vi "Copy Build to Shared Location.vi"(7 "Retain Build":bool, 8 "error in (no error)":errorcluster, 9 "Workspace":path, 10 "Job":string, 11 "Build Number":u32) -> (0 "error out":errorcluster)   [LabVIEW 2010]
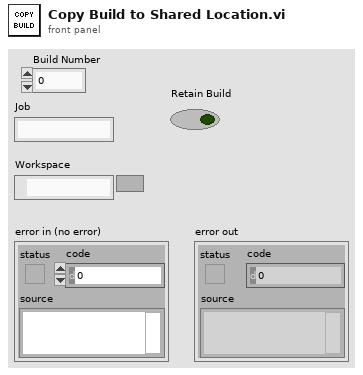
[diagram p1: front panel]
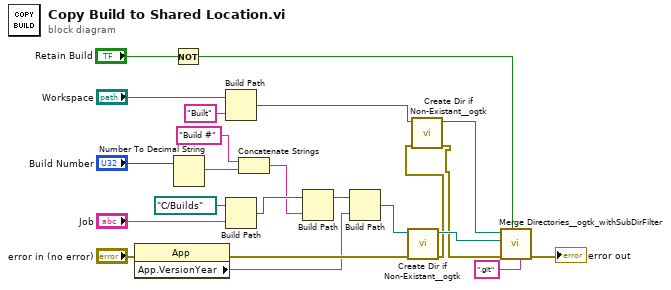
[diagram p0: block diagram]
diagram:
  n1 = property class="App"(error in="error in (no error)") -> (error out=w9:errorcluster, "App.VersionYear"=w7:string)  [unwired: 1 in, 1 out]
  n2 = Not(x="Retain Build") -> (.not. x?=w5:bool)
  n3 = Number To Decimal String(number="Build Number") -> (decimal integer string=w21:string)  [unwired: 1 in]
  n4 = Build Path(base path="Workspace", name or relative path="Built") -> (appended path=w4:path)
  n5 = Build Path(base path=path "C:/Builds", name or relative path="Job") -> (appended path=w20:path)
  n6 = Concatenate Strings("Build #", w21) -> (w8:string)
  n7 = Build Path(base path=w20, name or relative path=w8) -> (appended path=w10:path)
  n8 = Build Path(base path=w10, name or relative path=w7) -> (appended path=w19:path)
  n9 = call <userlib>:"Create Dir if Non-Existant__ogtk.vi"("error in (no error)"=w9, "Directory Path"=w19) -> ("error out"=w2:errorcluster, "dup Directory Path"=w15:path)  [unwired: 7 in, 1 out]
  n10 = call <userlib>:"Create Dir if Non-Existant__ogtk.vi"("error in (no error)"=w2, "Directory Path"=w4) -> ("error out"=w1:errorcluster, "dup Directory Path"=w3:path)  [unwired: 7 in, 1 out]
  n11 = call "Merge Directories__ogtk_withSubDirFilter.vi"("Subdir filter (\"\": none)"=".git" ("Subdir filter (\"\": none)"), "Delete Source? (FALSE)"=w5, "error in (no error)"=w1, "target directory path"=w15, "source directory path"=w3) -> ("error out"=→"error out":errorcluster)  [unwired: 5 in, 1 out]
